vi "Save Animated GIF Image (UTF-8 Path).vi"(6 "Animation Count (forever)":i32, 8 "error in (no error)":errorcluster, 9 "Delays":i32[](array[numeric]), 10 "Frames":T1[](array[typedef]), 11 "Path In":string) -> (0 "error out":errorcluster, 3 "Path Out":string)   [LabVIEW 2020, in "G-Image.lvlib"]
doc: "Saves a series of images in animated GIF format to disk.\n\nIf the input images have an alpha channel or mask, they will be used to set the transparent pixels of the resulting animated GIF.\n\n<b>Loop Count</b> sets the number of times the animation will play before looping, where 0 means loop forever."
uses:
  G-Image.lvlib
  <vilib>/picture/picture.llb/imagedata.ctl
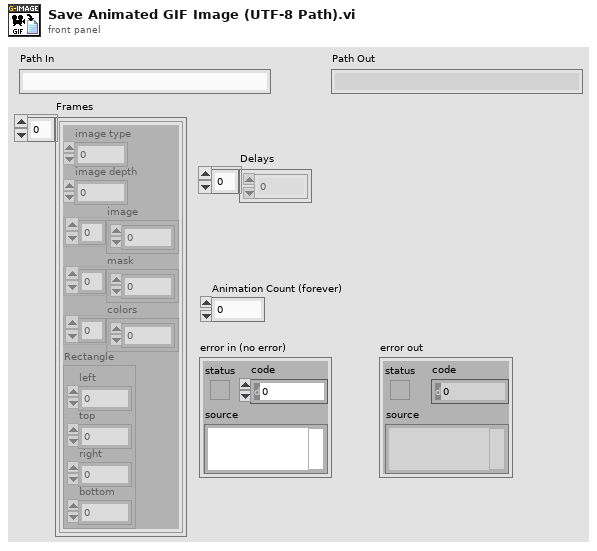
[diagram p1: front panel]
types:
  T1 = typedef "imagedata.ctl" = cluster{"image type":i32, "image depth":i32, "image":u8[], "mask":u8[], "colors":u32[], "Rectangle":cluster{"left":i16, "top":i16, "right":i16, "bottom":i16}}
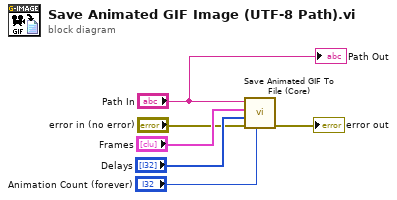
[diagram p0: block diagram]
diagram:
  n1 = call "Save Animated GIF To File (Core).vi"("Loop Count (forever)"="Animation Count (forever)", "error in (no error)"="error in (no error)", "Delays"="Delays", "Frames"="Frames", "Path In"="Path In") -> ("error out"=→"error out":errorcluster)  [unwired: 5 in, 1 out]
  "Path Out" <- "Path In"
